vi "Log My Data HDF5.vi"(4 "Data element":T3, 8 "error in":errorcluster, 11 "Refs":T1) -> (0 "error out":errorcluster, 3 "Refs out":T1)   [LabVIEW 2014]
uses:
  My Data HDF5 Refs.ctl
  <vilib>/UPVI/lvhdf5/library.llb/HDF5 Ref.ctl
  <vilib>/UPVI/lvhdf5/dataset.llb/Append Element(s) to Dataset (Variant).vi
  <vilib>/UPVI/lvhdf5/dataset.llb/Append Element(s) to Dataset.xnode
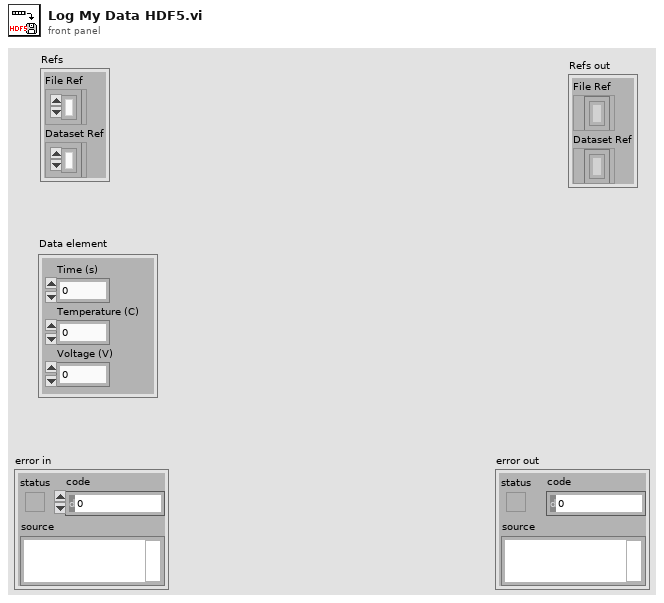
[diagram p1: front panel]
types:
  T1 = typedef "My Data HDF5 Refs.ctl" = cluster{"File Ref":T2, "Dataset Ref":T2}
  T2 = typedef "HDF5 Ref.ctl" = refnum<k1>
  T3 = cluster{"Time (s)":dbl, "Temperature (C)":dbl, "Voltage (V)":dbl}
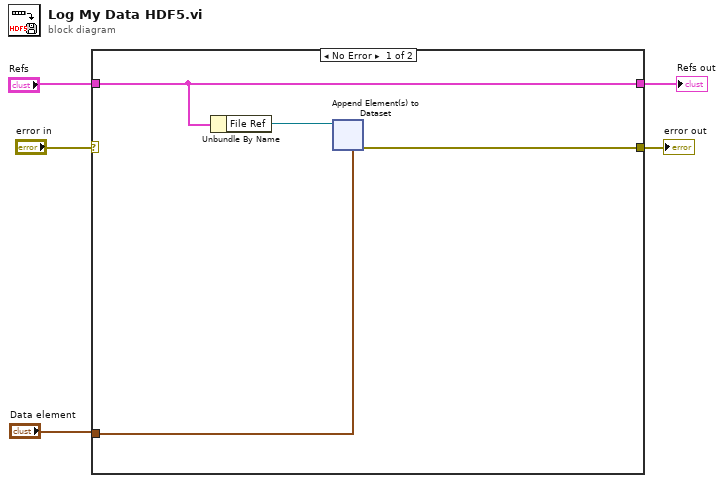
[diagram p0: block diagram]
diagram:
  n1 = case shown="No Error" "error in" {
    selector: "error in" -> [_ w19]
    tunnel: "Data element" -> [w6 _]
    tunnel: [w7 w19] -> w5
    tunnel: "Refs" -> [w9 w18]
    tunnel: [w9 w18] -> w1
    frame No Error {
      n2 = Unbundle By Name(w9) -> ("File Ref"=w8:T2)
      n3 = xnode "Append Element(s) to Dataset"("HDF5 Dataset Ref"=w8, "Data Element(s)"=w6) -> ("error out"=w7:errorcluster)  [unwired: 2 in, 3 out]
    }
    frame Error {
      # "Wire previous error through"
    }
  }
  "error out" <- w5
  "Refs out" <- w1
